vi "autoCoag.vi"(6 "Enum":T3, 8 "error in (no error)":errorcluster, 10 "data input":T2, 11 "setpoints":T1={"target clarified turbidity (NTU)"=0.3, "flocculator volume (L)"=0.0, "clarifier volume (L)"=0.0, "dose updates per HRT"=1} {"target clarified turbidity (NTU)" min=0.1 max=5.0 step=0.01; "dose updates per HRT" min=1 max=1000 step=1}) -> (0 "error out":errorcluster, 3 "setpoints out":T1 {"target clarified turbidity (NTU)" min=0.1 max=5.0 step=0.01; "dose updates per HRT" min=1 max=1000 step=1})   [LabVIEW 2019]
uses:
  state.ctl
  setpoints.ctl
  ProCoDA/DAQ configuration/Sensor buffer command.ctl
  data cluster.ctl
  calcDoseorGetGraph.ctl
  <vilib>/Utility/config.llb/Read Key (Double).vi
  <vilib>/Utility/config.llb/Read Key (U32).vi
  <vilib>/Utility/config.llb/Read Key (String).vi
  <vilib>/Utility/config.llb/Write Key (Double).vi
  <vilib>/Utility/config.llb/Write Key (U32).vi
  <vilib>/Utility/config.llb/Write Key (String).vi
  <vilib>/Utility/config.llb/NI_LVConfig.lvlib
panel:
  out "appended path":path
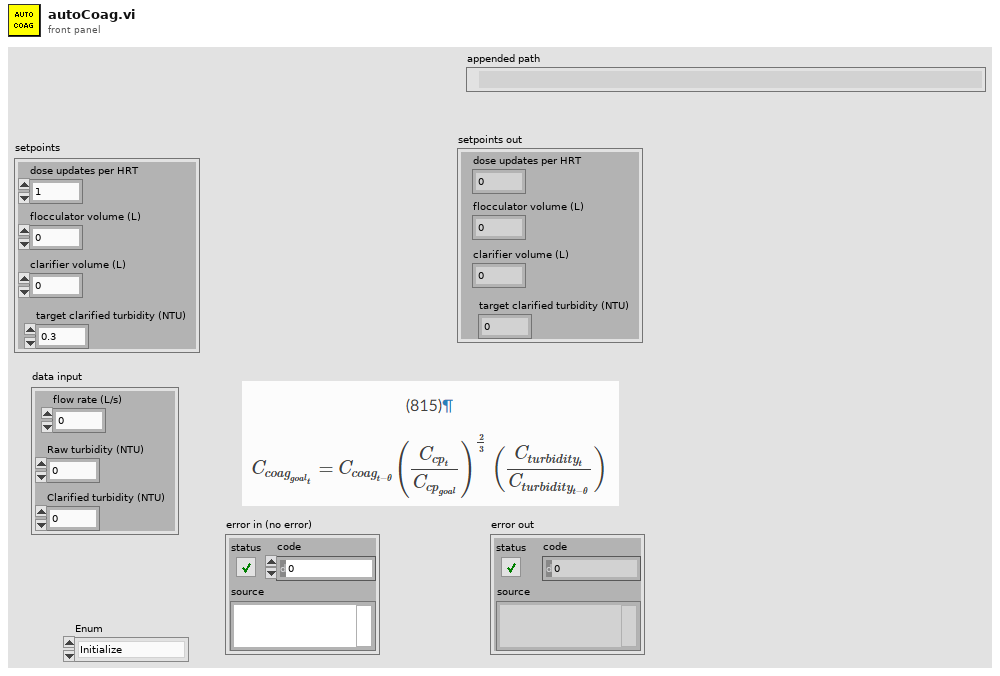
[diagram p1: front panel]
types:
  T1 = typedef "setpoints.ctl" = cluster{"target clarified turbidity (NTU)":dbl, "flocculator volume (L)":dbl, "clarifier volume (L)":dbl, "dose updates per HRT":u32}
  T2 = cluster{"Clarified turbidity (NTU)":dbl, "Raw turbidity (NTU)":dbl, "flow rate (L/s)":dbl}
  T3 = typedef "state.ctl" = enum16{"Initialize", "Change setpoints", "Process data", "Close"}
  T4 = typedef "Sensor buffer command.ctl" = enum16{"set buffer size", "write", "refill buffer", "read recent", "read all", "clear"}
  T5 = typedef "data cluster.ctl" = cluster{"Clarified turbidity (NTU)":dbl, "Raw turbidity (NTU)":dbl, "flow rate (L/s)":dbl, "time":timestamp}
  T6 = typedef "calcDoseorGetGraph.ctl" = enum16{"calculate dose", "read graph"}
  T7 = typedef "NI_LVConfig.lvlib/Config Data RefNum.ctl" = refnum<k1>
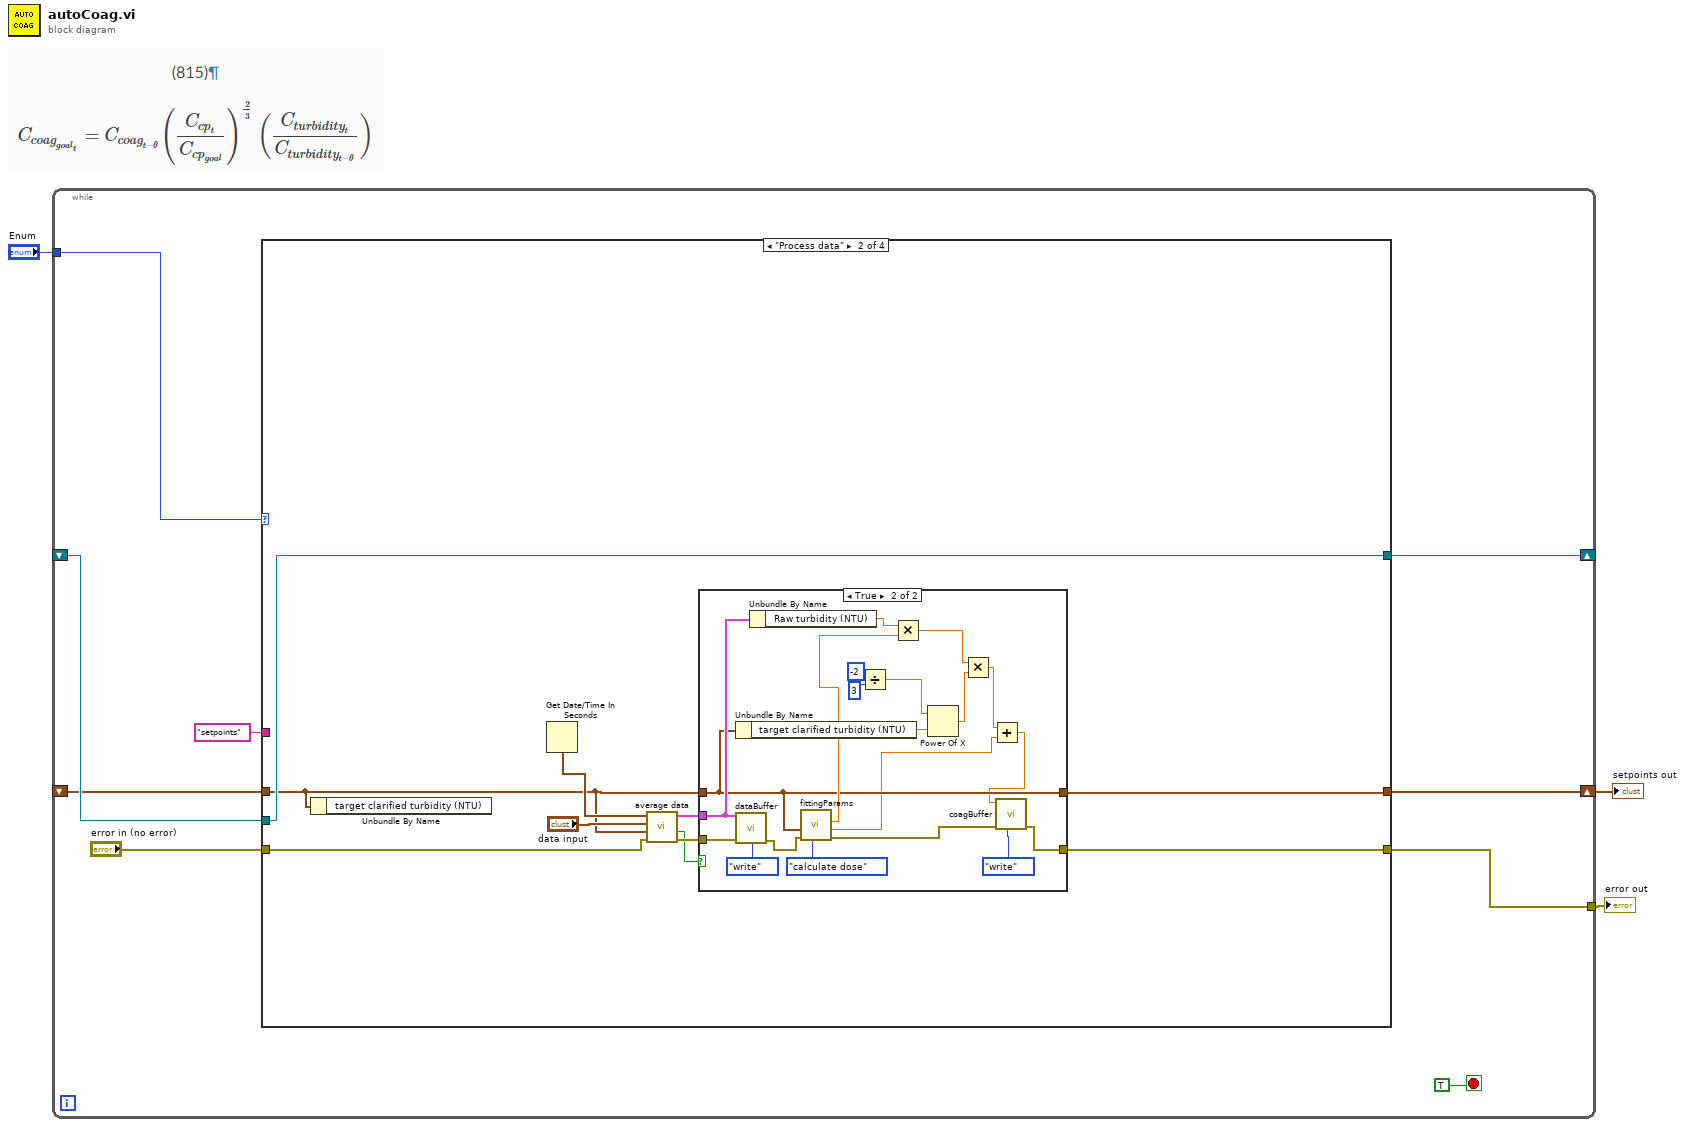
[diagram p0: block diagram]
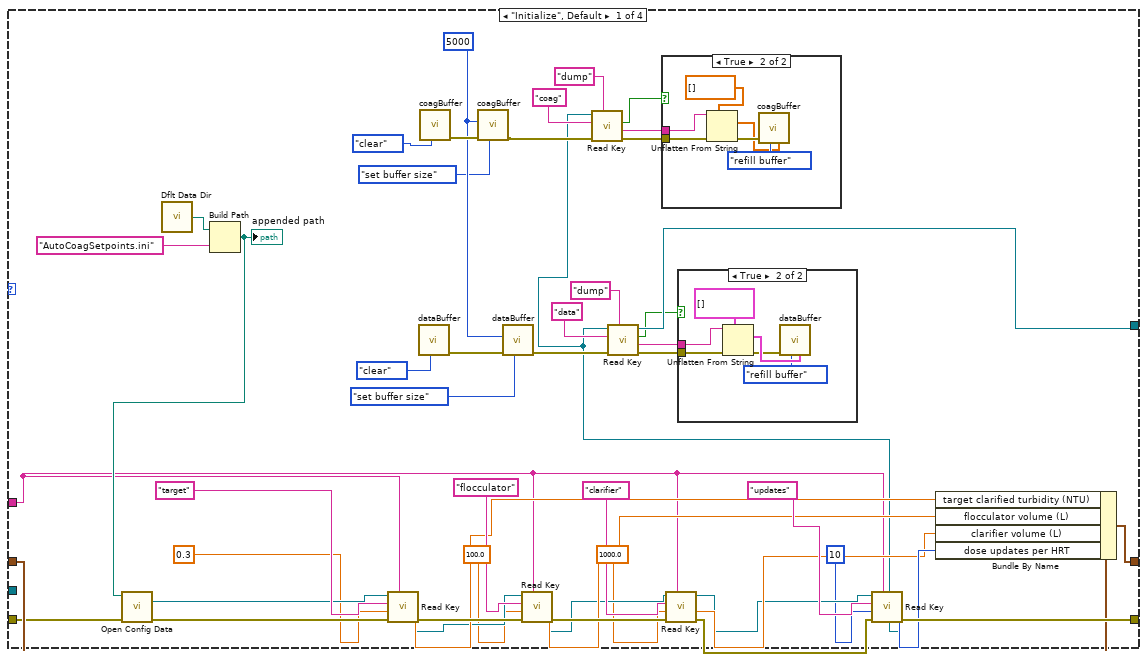
[diagram p2: hidden frame]
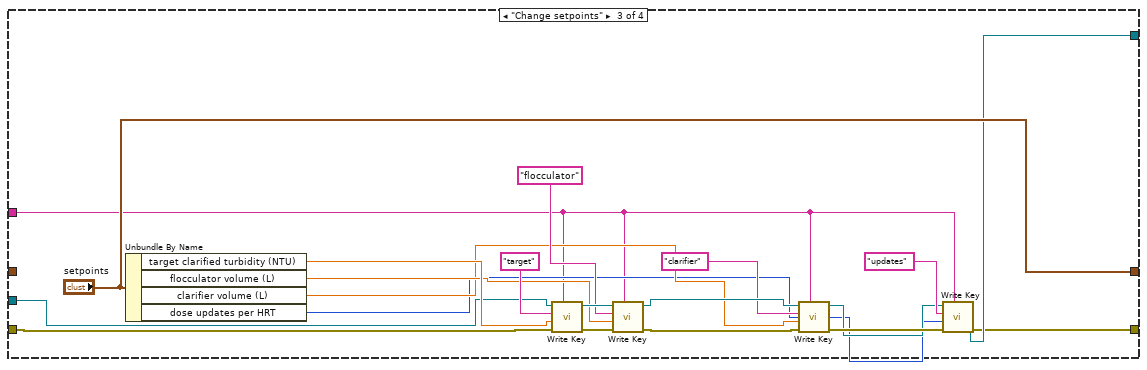
[diagram p6: hidden frame]
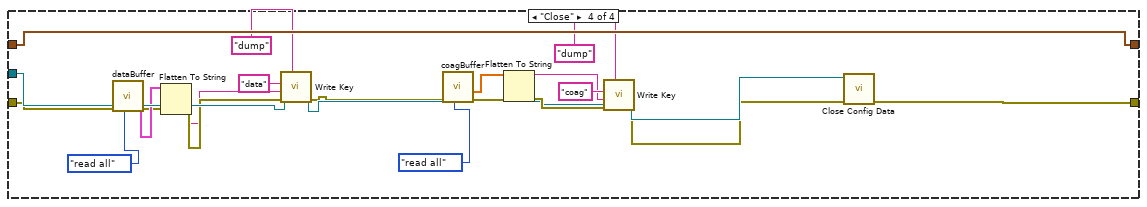
[diagram p7: hidden frame]
diagram:
  n1 = while {
    tunnel: "Enum" -> [w11]
    shift-right: [w10] -> w1
    shift-left: _ -> [w7]
    shift-right: [w9] -> _
    shift-left: _ -> [w8]
    tunnel: [w5] -> w2
    stop <- TRUE stop-if-true
    n2 = case shown="\"Process data\"" w11 {
      tunnel: [w49 w74 "setpoints" w146] -> w10
      tunnel: [w25 w83 w109 _] -> w9
      tunnel: w8 -> [_ w83 w110 w144]
      tunnel: w7 -> [w50 w75 _ w146]
      tunnel: "setpoints" ("section") -> [w40 _ w108 _]
      tunnel: [w51 w77 w107 w147] -> w5
      tunnel: "error in (no error)" -> [w35 w79 w106 w142]
      frame "Initialize", Default {
        w21 = u16 5000 ("max array size")
        n3 = call <vilib>:"Dflt Data Dir.vi"() -> ("App:Default Data Directory"=w34:path)
        n4 = Build Path(base path=w34, name or relative path="AutoCoagSetpoints.ini") -> (appended path=w60:path)
        "appended path" <- w60
        n5 = call <vilib>:"Open Config Data.vi"("error in (no error)"=w35, "configuration file path"=w60) -> ("error out"=w55:errorcluster, "refnum"=w44:T7)  [unwired: 7 in, 1 out]
        n6 = call-poly <vilib>:"Read Key.vi"("section"=w40, "error in (no error)"=w55, "default value"=0.3, "key"="target", "refnum"=w44) -> ("error out"=w54:errorcluster, "value"=w45:dbl, "refnum out"=w43:T7)  [unwired: 3 in, 1 out]
        n7 = call "dataBuffer.vi"("command"=Sensor_buffer_command."clear") -> ("error out"=w31:errorcluster)  [unwired: 8 in, 2 out]
        n8 = call "coagBuffer.vi"("command"=Sensor_buffer_command."clear") -> ("error out"=w22:errorcluster)  [unwired: 8 in, 2 out]
        n9 = call "coagBuffer.vi"("command"=Sensor_buffer_command."set buffer size", "error in (no error)"=w22, "max array size"=w21) -> ("error out"=w14:errorcluster)  [unwired: 6 in, 2 out]
        n10 = call "dataBuffer.vi"("command"=Sensor_buffer_command."set buffer size", "error in (no error)"=w31, "max array size"=w21) -> ("error out"=w28:errorcluster)  [unwired: 6 in, 2 out]
        n11 = call-poly <vilib>:"Read Key.vi"("section"=w40, "error in (no error)"=w54, "default value"=100.0, "key"="flocculator", "refnum"=w43) -> ("error out"=w53:errorcluster, "value"=w46:dbl, "refnum out"=w42:T7)  [unwired: 3 in, 1 out]
        n12 = call-poly <vilib>:"Read Key.vi"("section"=w40, "error in (no error)"=w53, "default value"=1000.0, "key"="clarifier", "refnum"=w42) -> ("error out"=w52:errorcluster, "value"=w47:dbl, "refnum out"=w41:T7)  [unwired: 3 in, 1 out]
        n13 = call-poly <vilib>:"Read Key.vi"("section"=w40, "error in (no error)"=w52, "default value"=u32 10, "key"="updates", "refnum"=w41) -> ("error out"=w51:errorcluster, "value"=w48:u32, "refnum out"=w13:T7)  [unwired: 3 in, 1 out]
        n14 = call-poly <vilib>:"Read Key.vi"("section"="dump", "error in (no error)"=w14, "key"="coag", "refnum"=w13) -> ("error out"=w17:errorcluster, "value"=w18:string, "found?"=w19:bool)  [unwired: 4 in, 1 out]
        n15 = call-poly <vilib>:"Read Key.vi"("section"="dump", "error in (no error)"=w28, "key"="data", "refnum"=w13) -> ("error out"=w27:errorcluster, "value"=w26:string, "found?"=w24:bool, "refnum out"=w25:T7)  [unwired: 4 in]
        n16 = case shown="True" w19 {
          tunnel: w17 -> [_ w67]
          tunnel: w18 -> [_ w66]
          frame False {
          }
          frame True {
            n17 = Unflatten From String(type=dbl[] [] ("all coag out"), binary string=w66, error in (no error)=w67) -> (value=w62:dbl[], error out=w64:errorcluster)  [unwired: 2 in, 1 out]
            n18 = call "coagBuffer.vi"("all coag in"=w62, "command"=Sensor_buffer_command."refill buffer", "error in (no error)"=w64) -> ()  [unwired: 6 in, 3 out]
          }
        }
        n19 = case shown="True" w24 {
          tunnel: w27 -> [_ w73]
          tunnel: w26 -> [_ w72]
          frame False {
          }
          frame True {
            n20 = Unflatten From String(type=T5[] [] ("all data out"), binary string=w72, error in (no error)=w73) -> (value=w70:T5[], error out=w68:errorcluster)  [unwired: 2 in, 1 out]
            n21 = call "dataBuffer.vi"("all data in"=w70, "command"=Sensor_buffer_command."refill buffer", "error in (no error)"=w68) -> ()  [unwired: 6 in, 3 out]
          }
        }
        n22 = Bundle By Name(cluster=w50, "target clarified turbidity (NTU)"=w45, "flocculator volume (L)"=w46, "clarifier volume (L)"=w47, "dose updates per HRT"=w48) -> (w49:T1)
      }
      frame "Process data" {
        n23 = Unbundle By Name(w75) -> ()  [unwired: 1 out]
        n24 = Get Date/Time In Seconds() -> (seconds since 1Jan1904=w81:timestamp)
        n25 = call "average data.vi"("error in (no error)"=w79, "setpoints"=w75, "data input"="data input", "seconds since 1Jan1904"=w81) -> ("error out"=w78:errorcluster, "new interval"=w76:bool, "averaged data"=w80:T5)  [unwired: 5 in]
        n26 = case shown="True" w76 {
          tunnel: w80 -> [_ w101]
          tunnel: w78 -> [w85 w104]
          tunnel: [w85 w87] -> w77
          tunnel: w75 -> [w84 w98]
          tunnel: [w84 w98] -> w74
          frame False {
          }
          frame True {
            n27 = Unbundle By Name(w98) -> ("target clarified turbidity (NTU)"=w97:dbl)
            n28 = call "dataBuffer.vi"("command"=Sensor_buffer_command."write", "error in (no error)"=w104, "averaged data"=w101) -> ("error out"=w103:errorcluster)  [unwired: 6 in, 2 out]
            n29 = Unbundle By Name(w101) -> ("Raw turbidity (NTU)"=w100:dbl)
            n30 = call "fittingParams.vi"("read/write"=calcDoseorGetGraph."calculate dose", "error in (no error)"=w103, "setpoints"=w98) -> ("error out"=w89:errorcluster, "Ccoag-DOM"=w90:dbl, "Ku*"=w99:dbl)  [unwired: 4 in, 1 out]
            n31 = Divide(x=-2, y=3) -> (x/y=w94:dbl)
            n32 = Multiply(x=w100, y=w99) -> (x*y=w93:dbl)
            n33 = Power Of X(1:w97, 2:w94) -> (0:w92:dbl)
            n34 = Multiply(x=w93, y=w92) -> (x*y=w91:dbl)
            n35 = Add(x=w91, y=w90) -> (x+y=w88:dbl)
            n36 = call "coagBuffer.vi"("command"=Sensor_buffer_command."write", "error in (no error)"=w89, "Coag dose"=w88) -> ("error out"=w87:errorcluster)  [unwired: 6 in, 2 out]
          }
        }
      }
      frame "Change setpoints" {
        n37 = Unbundle By Name("setpoints") -> ("target clarified turbidity (NTU)"=w115:dbl, "flocculator volume (L)"=w114:dbl, "clarifier volume (L)"=w113:dbl, "dose updates per HRT"=w112:u32)
        n38 = call-poly <vilib>:"Write Key.vi"("section"=w108, "error in (no error)"=w106, "value"=w115, "key"="target", "refnum"=w110) -> ("error out"=w124:errorcluster, "refnum out"=w122:T7)  [unwired: 4 in, 1 out]
        n39 = call-poly <vilib>:"Write Key.vi"("section"=w108, "error in (no error)"=w124, "value"=w114, "key"="flocculator", "refnum"=w122) -> ("error out"=w123:errorcluster, "refnum out"=w121:T7)  [unwired: 4 in, 1 out]
        n40 = call-poly <vilib>:"Write Key.vi"("section"=w108, "error in (no error)"=w123, "value"=w113, "key"="clarifier", "refnum"=w121) -> ("error out"=w117:errorcluster, "refnum out"=w116:T7)  [unwired: 4 in, 1 out]
        n41 = call-poly <vilib>:"Write Key.vi"("section"=w108, "error in (no error)"=w117, "value"=w112, "key"="updates", "refnum"=w116) -> ("error out"=w107:errorcluster, "refnum out"=w109:T7)  [unwired: 4 in, 1 out]
      }
      frame "Close" {
        n42 = call "dataBuffer.vi"("command"=Sensor_buffer_command."read all", "error in (no error)"=w142) -> ("error out"=w141:errorcluster, "all data out"=w143:T5[])  [unwired: 7 in, 1 out]
        n43 = Flatten To String(anything=w143, error in (no error)=w141) -> (data string=w139:string, error out=w140:errorcluster)  [unwired: 2 in, 1 out]
        n44 = call-poly <vilib>:"Write Key.vi"("section"="dump", "error in (no error)"=w140, "value"=w139, "key"="data", "refnum"=w144) -> ("error out"=w127:errorcluster, "refnum out"=w129:T7)  [unwired: 4 in, 1 out]
        n45 = call "coagBuffer.vi"("command"=Sensor_buffer_command."read all", "error in (no error)"=w127) -> ("error out"=w134:errorcluster, "all coag out"=w135:dbl[])  [unwired: 7 in, 1 out]
        n46 = Flatten To String(anything=w135, error in (no error)=w134) -> (data string=w131:string, error out=w130:errorcluster)  [unwired: 2 in, 1 out]
        n47 = call-poly <vilib>:"Write Key.vi"("section"="dump", "error in (no error)"=w130, "value"=w131, "key"="coag", "refnum"=w129) -> ("error out"=w126:errorcluster, "refnum out"=w128:T7)  [unwired: 4 in, 1 out]
        n48 = call <vilib>:"Close Config Data.vi"("error in (no error)"=w126, "refnum"=w128) -> ("error out"=w147:errorcluster)  [unwired: 8 in, 1 out]
      }
    }
  }
  "error out" <- w2
  "setpoints out" <- w1
